vi "AM Start test.vi"(8 "error in (no error)":errorcluster, 9 "Variant":variant, 10 "Message Queues in":T1, 11 "Hardware Resources in":T2 {"PS Measure Plan" items=["Pretreatment settings (PS)", "Linear Sweep Voltammetry (LSV)", "Differential Pulse Voltammetry (DPV)", "Cyclic Voltammetry (CV)", "Chronoamperometry (CA)", "Chronopotentiometry (CP)", "El Imp Spectroscopy (EIS)"]; "System Preset"."Test Configuration"."SP List" format="%#.1g"}) -> (0 "error out":errorcluster, 3 "Hardware Resources out":T2 {"PS Measure Plan" items=["Pretreatment settings (PS)", "Linear Sweep Voltammetry (LSV)", "Differential Pulse Voltammetry (DPV)", "Cyclic Voltammetry (CV)", "Chronoamperometry (CA)", "Chronopotentiometry (CP)", "El Imp Spectroscopy (EIS)"]; "System Preset"."Test Configuration"."SP List" format="%#.1g"})   [LabVIEW 2020, in "Test Driver.lvlib"]
doc: "Configure the hardware."
uses:
  Test Driver.lvlib
  Test Driver Configuration.ctl
  support/Message Queue/Message Cluster.ctl
  System Preset.ctl
  Test Type.ctl
  support/Message Queue/All Message Queues.ctl
  support/Message Queue/Enqueue Message (Single).vi
  support/Message Queue/Message Queue.lvlib
panel:
  # "X"
  # "Y"
  # "Cycles"
  # "Point Delay"
  # "Up"
  # "Down"
  # "Z Axes"
  # "#C"
  # "In"
  # "Out"
  # "Cleaning [sec]"
  # "X"
  # "Y"
  # "Cycles"
  # "Point Delay"
  # "Up"
  # "Down"
  # "Z Axes"
  # "#C"
  # "In"
  # "Out"
  # "Cleaning [sec]"
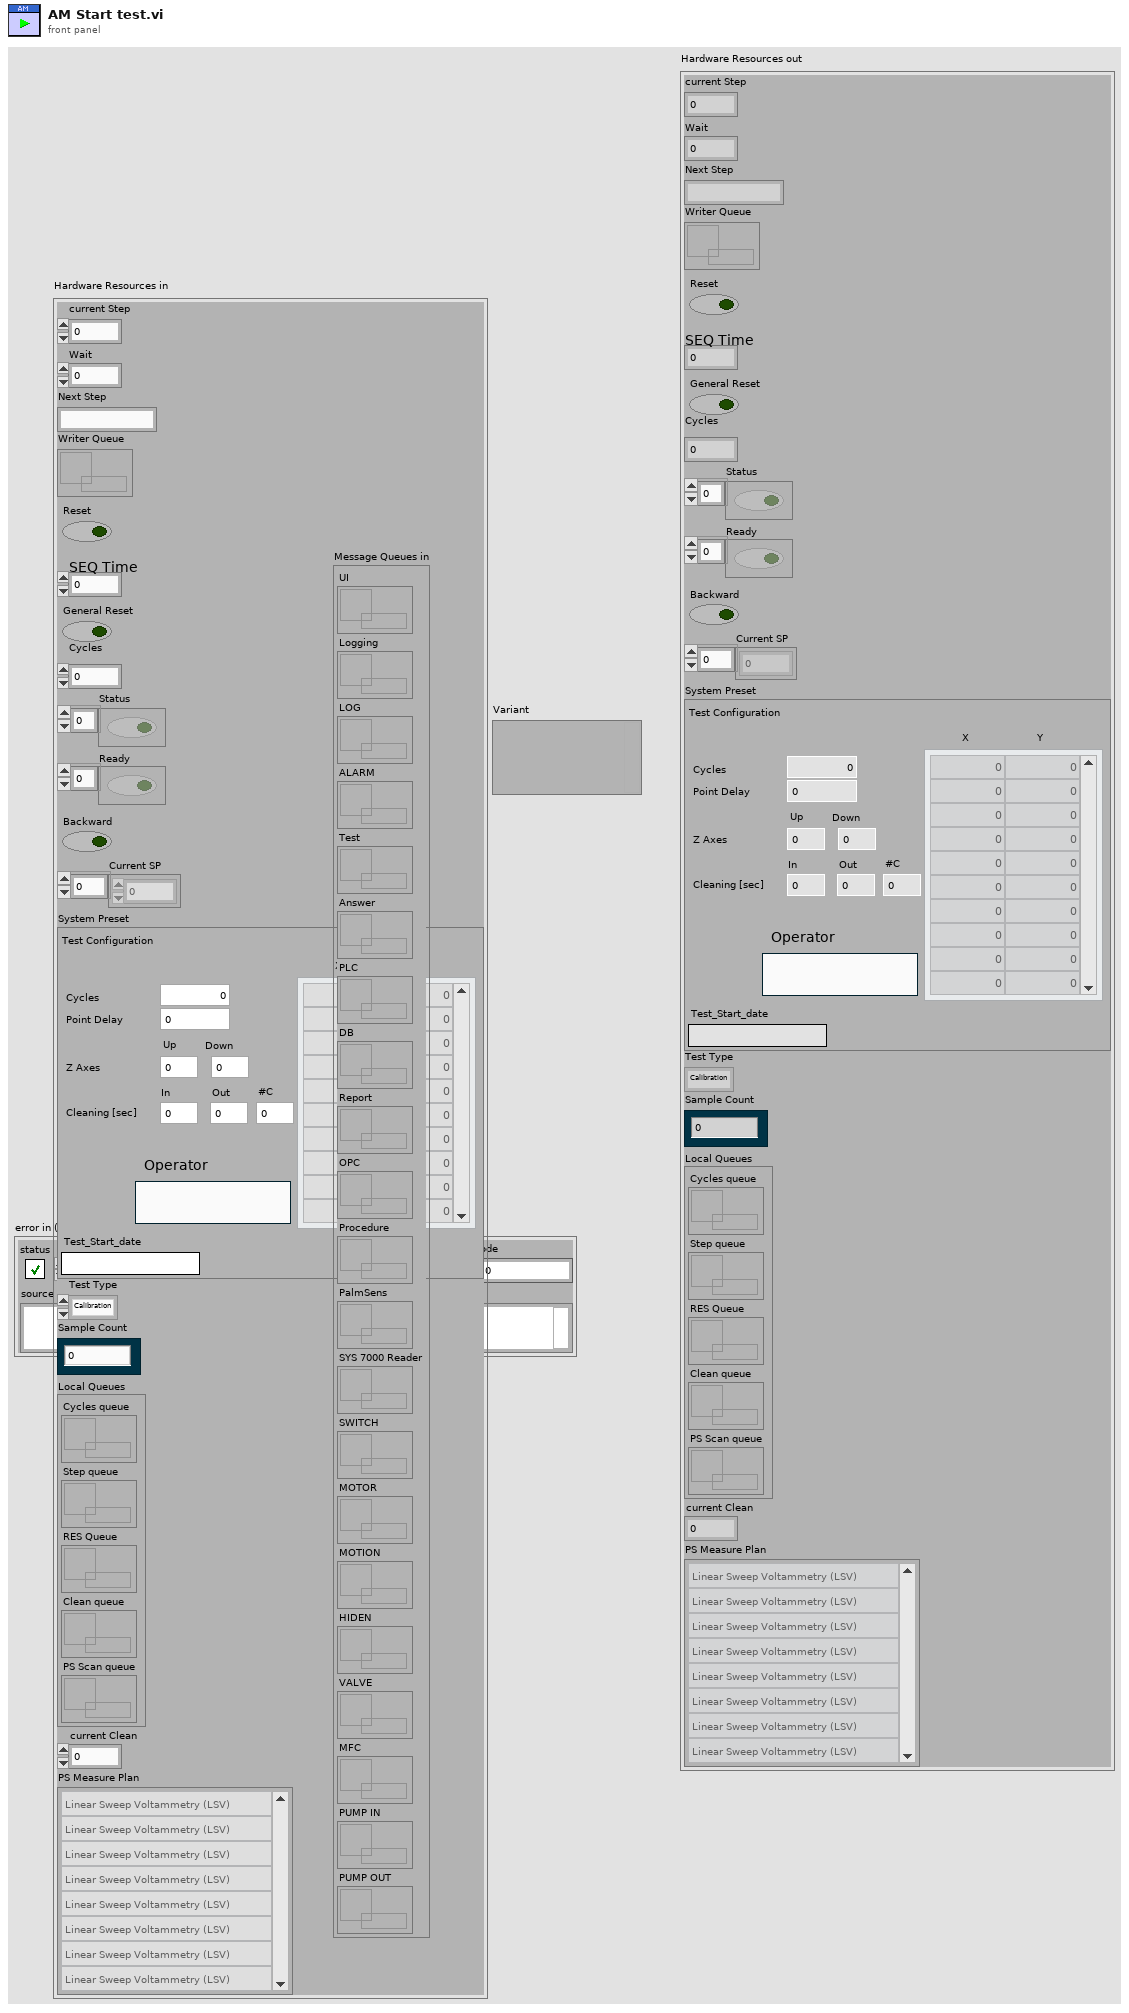
[diagram p1: front panel]
types:
  T1 = typedef "Message Queue.lvlib/All Message Queues.ctl" = cluster{"UI":refnum<queue>, "Logging":refnum<queue>, "LOG":refnum<queue>, "ALARM":refnum<queue>, "Test":refnum<queue>, "Answer":refnum<queue>, "PLC":refnum<queue>, "DB":refnum<queue>, "Report":refnum<queue>, "OPC":refnum<queue>, "Procedure":refnum<queue>, "PalmSens":refnum<queue>, "SYS 7000 Reader":refnum<queue>, "SWITCH":refnum<queue>, "MOTOR":refnum<queue>, "MOTION":refnum<queue>, "HIDEN":refnum<queue>, "VALVE":refnum<queue>, "MFC":refnum<queue>, "PUMP IN":refnum<queue>, "PUMP OUT":refnum<queue>}
  T2 = typedef "Test Driver.lvlib/Test Driver Configuration.ctl" = cluster{"current Step":i32, "Wait":dbl, "Next Step":string, "Writer Queue":refnum<queue>, "Reset":bool, "SEQ Time":i32, "General Reset":bool, "Cycles":i32, "Status":bool[], "Ready":bool[], "Backward":bool, "Current SP":dbl[], "System Preset":T3, "Test Type":T4, "Sample Count":i32, "Local Queues":cluster{"Cycles queue":refnum<queue>, "Step queue":refnum<queue>, "RES Queue":refnum<queue>, "Clean queue":refnum<queue>, "PS Scan queue":refnum<queue>}, "current Clean":i32, "PS Measure Plan":u16[]}
  T3 = typedef "System Preset.ctl" = cluster{"Test Configuration":cluster{"Cycles":i32, "Z Up":dbl, "SP List":dbl[][], "Operator":string, "Point Delay":i32, "Z Up 2":dbl, "Cleaning In":dbl, "Cleaning Out":dbl, "Cleaning Cycles":i32}, "Test_Start_date":string}
  T4 = typedef "Test Driver.lvlib/Test Type.ctl" = enum16{"Calibration", "Test"}
  T5 = cluster{"Type CMD":string, "Mode CMD":string, "Main CMD":string}
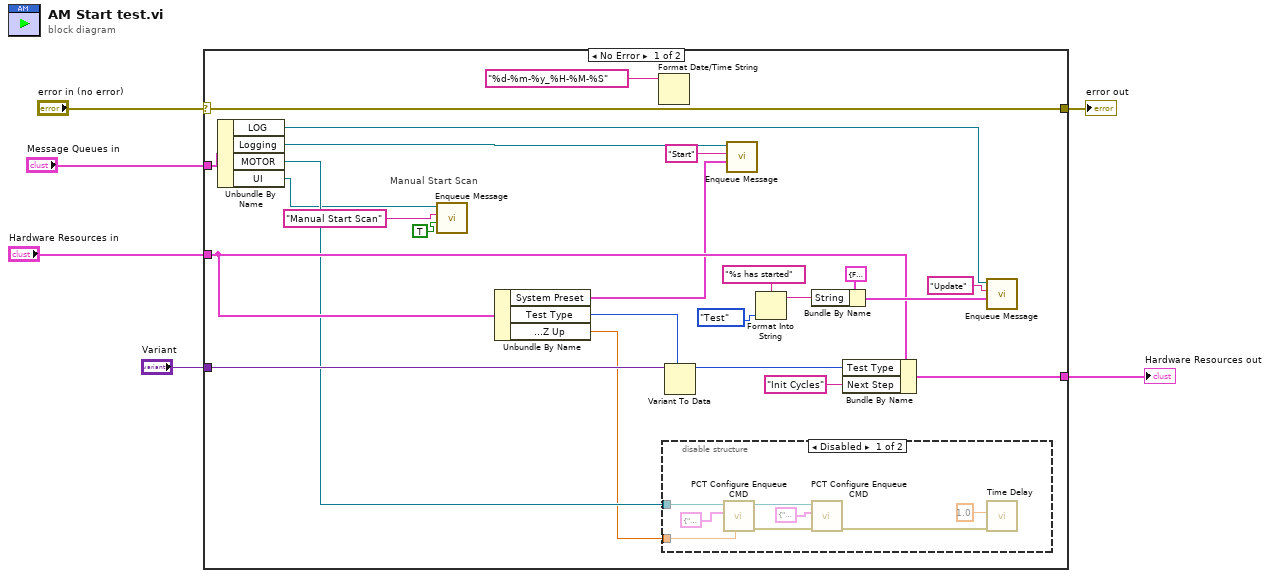
[diagram p0: block diagram]
diagram:
  n1 = case shown="No Error" "error in (no error)" {
    selector: "error in (no error)" -> [w30 w39]
    tunnel: [w30 w39] -> w5
    tunnel: "Hardware Resources in" -> [w17 w40]
    tunnel: [w27 w40] -> w3
    tunnel: "Message Queues in" -> [w24 _]
    tunnel: "Variant" -> [w29 _]
    frame No Error {
      # "Manual Start Scan"
      n2 = Unbundle By Name(w24) -> ("LOG"=w13:refnum<queue>, "Logging"=w20:refnum<queue>, "MOTOR"=w14:refnum<queue>, "UI"=w9:refnum<queue>)
      n3 = call-poly "Enqueue Message.vi"("Message Data"=TRUE, "Message"="Manual Start Scan", "Message Queue"=w9) -> ()  [unwired: 7 in, 2 out]
      n4 = Unbundle By Name(w17) -> ("System Preset"=w15:T3, "Test Type"=w28:T4, "System Preset.Test Configuration.Z Up"=w12:dbl)
      n5 = Format Date/Time String(time format string (%c)="%d-%m-%y_%H-%M-%S") -> ()  [unwired: 2 in, 1 out]
      n6 = disable-structure shown="Disabled" {
        disable-tunnel: w14 -> [w33 _]
        disable-tunnel: w12 -> [w32 _]
        frame Disabled {
          n7 = call "PCT Configure Enqueue CMD.vi"("Parameter Data"=w32, "CMD"=T5 {"Type CMD"="Speed", "Mode CMD"="", "Main CMD"="Configure"}, "CMD Queue in"=w33) -> ("error out"=w31:errorcluster, "CMD Queue out"=w37:refnum<queue>)  [unwired: 6 in, 1 out]
          n8 = call "PCT Configure Enqueue CMD.vi"("error in (no error)"=w31, "CMD"=T5 {"Type CMD"="Reset", "Mode CMD"="Counter", "Main CMD"="Utility"}, "CMD Queue in"=w37) -> ("error out"=w36:errorcluster)  [unwired: 6 in, 2 out]
          n9 = call "Time Delay"("error in (no error)"=w36, "Delay Time (s)"=1.0) -> ()  [unwired: 9 in, 1 out]
        }
        frame Enabled {
        }
      }
      n10 = Variant To Data(type=w28, Variant=w29) -> (data=w19:T4)  [unwired: 1 in, 1 out]
      n11 = call-poly "Enqueue Message.vi"("Message Data"=w15, "Message"="Start", "Message Queue"=w20) -> ()  [unwired: 7 in, 2 out]
      n12 = Format Into String(format string="%s has started", Test_Type."Test" ("data")) -> (resulting string=w22:string)  [unwired: 2 in, 1 out]
      n13 = Bundle By Name(cluster=cluster{"Replace":bool, "String":string} {"Replace"=FALSE, "String"="Procedure was started"}, "String"=w22) -> (w23:cluster{"Replace":bool, "String":string})
      n14 = Bundle By Name(cluster=w17, "Test Type"=w19, "Next Step"="Init Cycles" ("Message")) -> (w27:T2)
      n15 = call-poly "Enqueue Message.vi"("Message Data"=w23, "Message"="Update" ("Main CMD"), "Message Queue"=w13) -> ()  [unwired: 7 in, 2 out]
    }
    frame Error {
    }
  }
  "Hardware Resources out" <- w3
  "error out" <- w5
